vi "global config.vi"() -> ()   [LabVIEW 2011]
uses:
  chanel.ctl
  signal type.ctl
  gain.ctl
  single chanel.ctl
  CARD config.ctl
  chanelconfig/filter.ctl
  chanelconfig/Power_config.ctl
  sort/CHsort index.ctl
  display_subvi/cH display.ctl
panel:
  out "tempt index":T2(array[cluster]) {"Car"."CH dispaly"."multi" min=0.0}
  out "chart index":T2(array[cluster]) {"Car"."CH dispaly"."multi" min=0.0}
  out "display indexout":T3(array[cluster]) {"Car"."CH dispaly"."multi" min=0.0}
  out "display config":cluster{"CH dispaly":T1, "card":i32, "ch":i32}[](array[cluster]) {"CH dispaly"."multi" min=0.0}
  out "CARD k&B ARRAY":T4(array[cluster])
  out "card sort":cluster{"sort Array":T5[]}[](array[cluster])
  out "sort table out":cluster{"table data":string[][], "length":u16}[](array[cluster])
  in  "DisplayIndexConfig":T6(array[cluster])
  in  "sensor":T7(array[cluster])
  in  "all device":T8
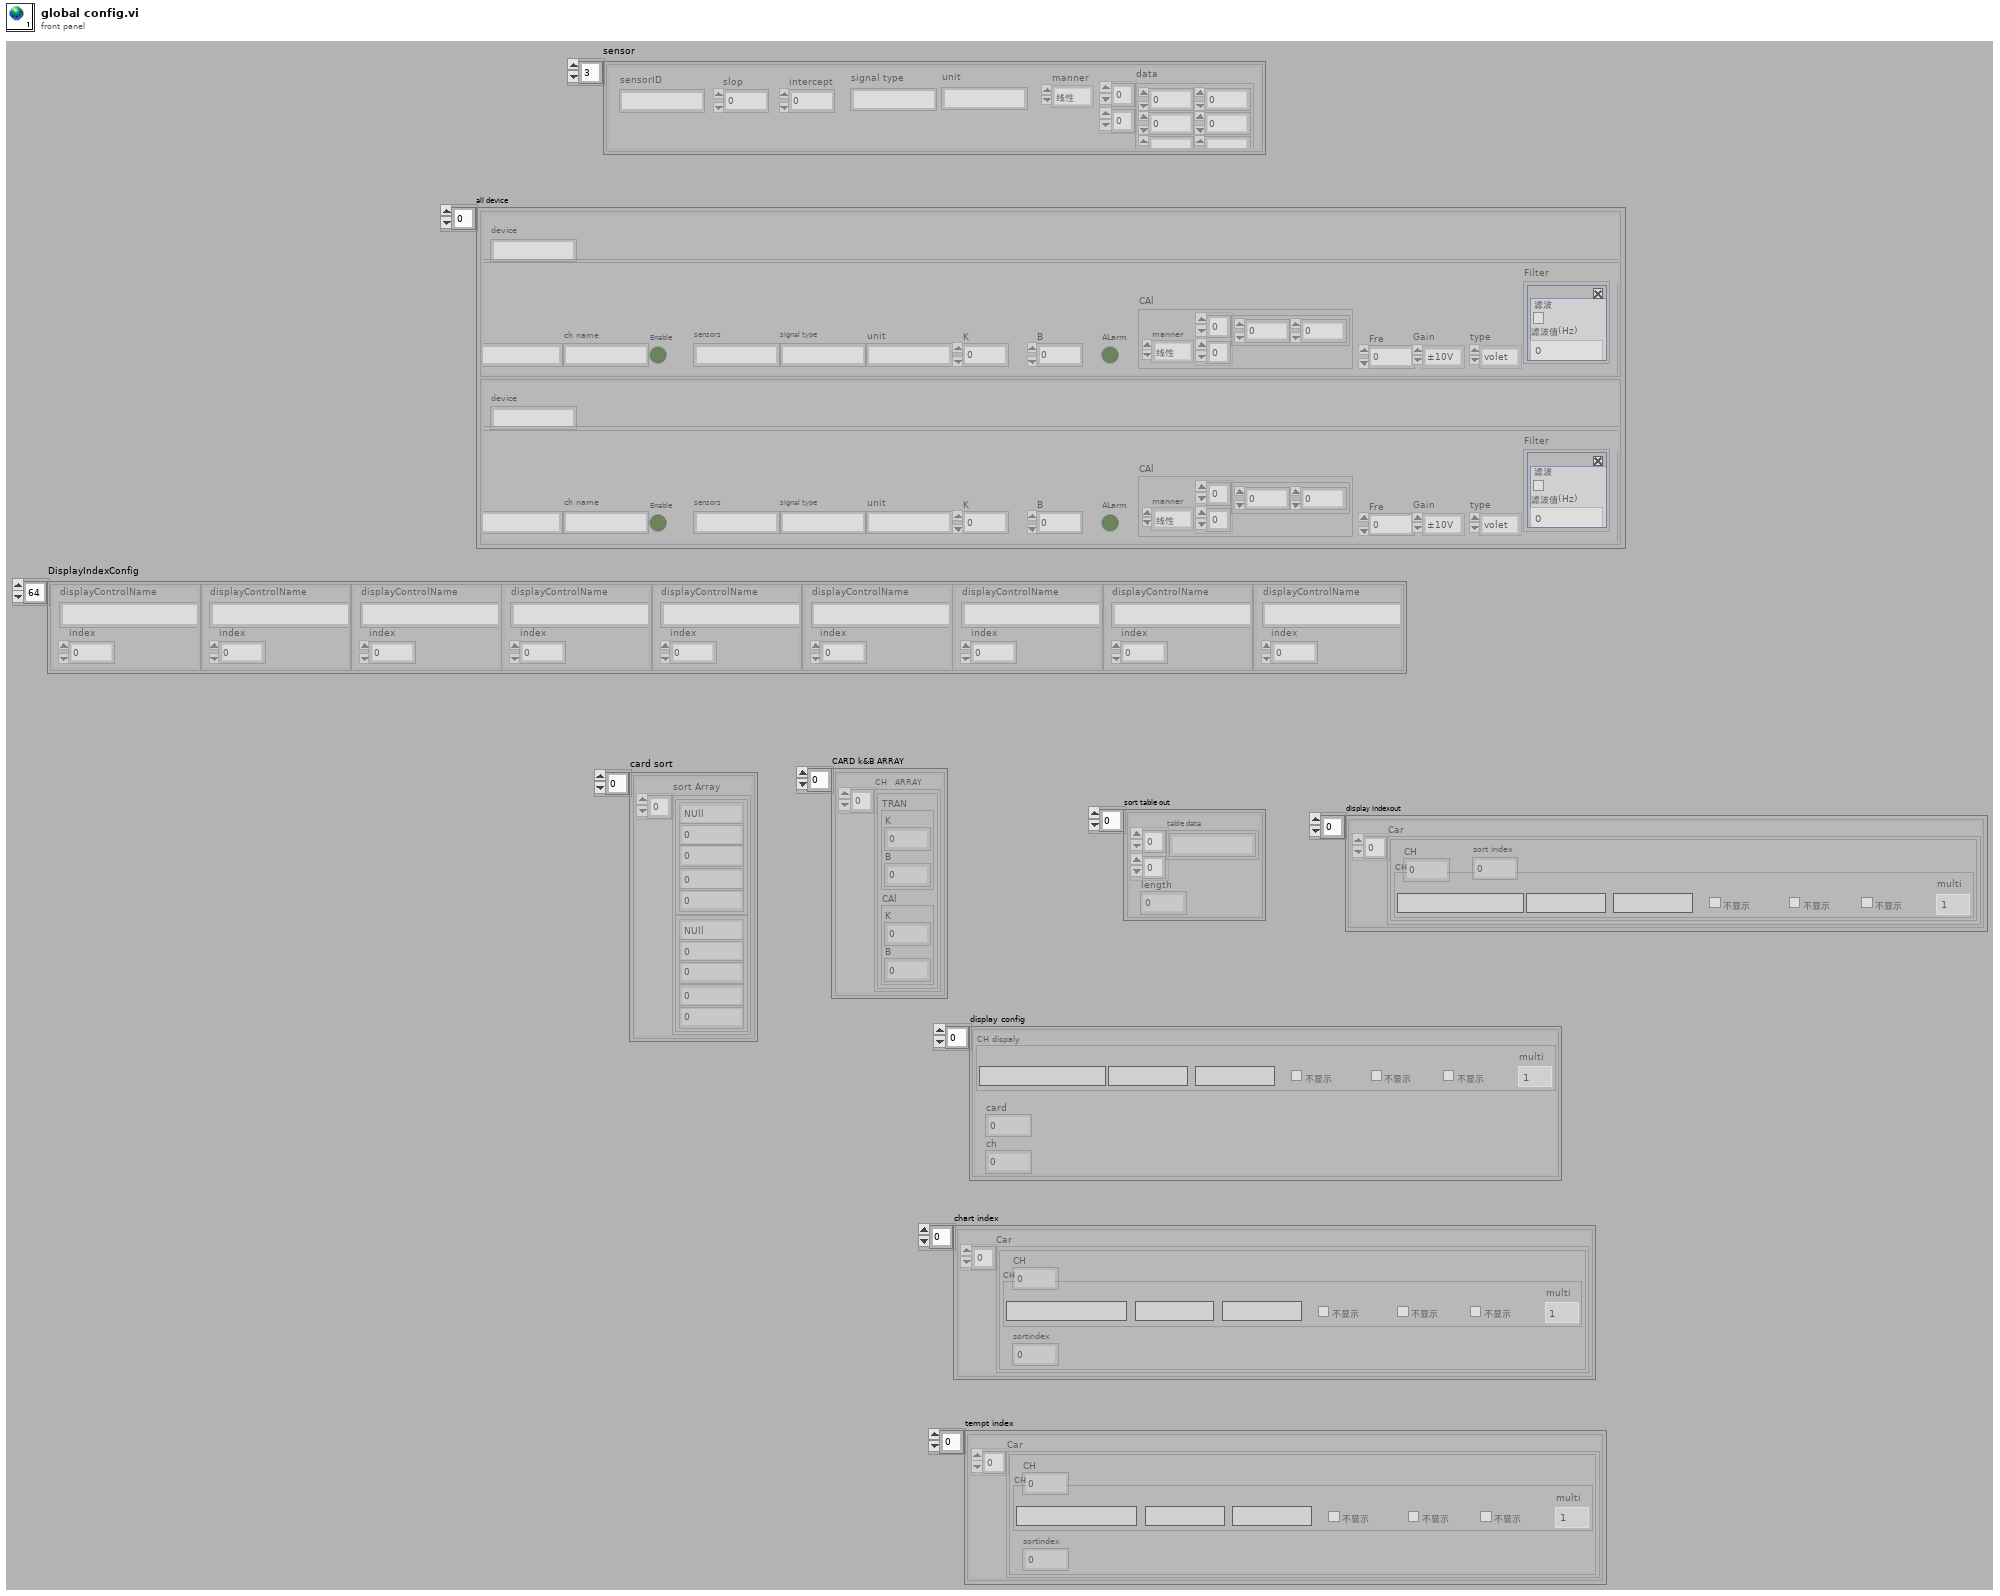
[diagram p1: front panel]
types:
  T1 = typedef "cH display.ctl" = cluster{"Name":string, "list":bool, "chart":bool, "signal type":string, "unit":string, "tempt":bool, "multi":dbl}
  T2 = cluster{"Car":cluster{"CH":i32, "CH dispaly":T1, "sortindex":i32}[]}[]
  T3 = cluster{"Car":cluster{"CH":i32, "CH dispaly":T1, "sort index":i32}[]}[]
  T4 = cluster{"CH　ARRAY":cluster{"TRAN":cluster{"K":sgl, "B":sgl}, "CAl":cluster{"K":sgl, "B":sgl}}[]}[]
  T5 = typedef "CHsort index.ctl" = cluster{"sort":enum16{"NUll", "Vibration", "IN DATA", "IN I", "IN T", "OUT DATA", "OUT I", "L"}, "index":i32, "length":i32, "sort index":i32, "sort length":i32}
  T6 = cluster{"displayControlName":string, "index":i32}[]
  T7 = cluster{"manner":enum16{"线性", "查表"}, "data":dbl[][], "slop":dbl, "intercept":dbl, "sensorID":string, "signal type":string, "unit":string}[]
  T8 = typedef "chanel.ctl" = T9[]
  T9 = typedef "CARD config.ctl" = cluster{"device":string, "ch":T10[]}
  T10 = typedef "single chanel.ctl" = cluster{"chanel":string, "ch name":string, "Enable":bool, "sensors":string, "signal type":string, "unit":string, "K":dbl, "B":dbl, "ALarm":bool, "CAl":cluster{"manner":enum16{"线性", "查表"}, "data":dbl[][]}, "Fre":dbl, "type":T11, "Gain":T12, "Filter":T13, "Power":T14}
  T11 = typedef "signal type.ctl" = enum16{"未设置", "volet", "current", "vibration", "electric charge ", "resistance "}
  T12 = typedef "gain.ctl" = enum16{"±10V", "±5V", "±2.5V", "±1V", "±500mV", "±100mV", "10V", "5V", "2.5V", "1V", "500mV", "100mV"}
  T13 = typedef "filter.ctl" = cluster{"en":bool, "value":i32, "Boolean":bool}
  T14 = typedef "Power_config.ctl" = cluster{"power_en":bool, "Mode":enum16{"电压", "电流"}, "value":dbl, "Boolean":bool}
diagram:
